vi "AcquireHardware2.vi"(8 "error in (no error)":errorcluster, 11 "SkySparkDevice in":refnum<class "SkySparkDevice.lvclass">) -> (0 "error out":errorcluster, 3 "SkySparkDevice out":refnum<class "SkySparkDevice.lvclass">)   [LabVIEW 2020, in "SkySparkDevice.lvclass"]
uses:
  SkySparkDevice.lvclass
  FGVFunctionTypeDef.ctl
  FGV_TypeDef.ctl
  SkySparkDevice.lvclass/SkySparkDevice.ctl
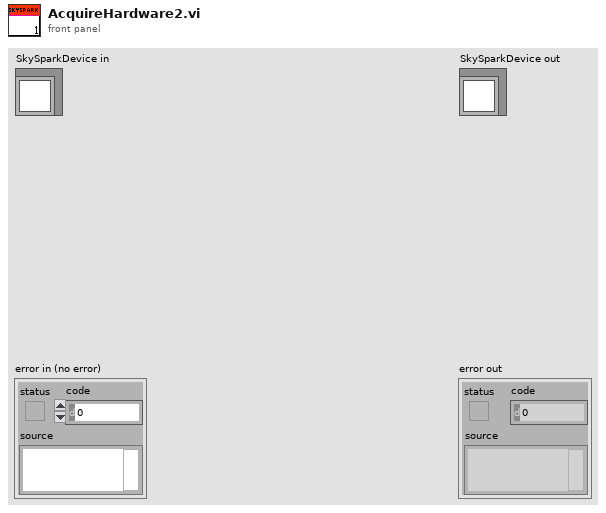
[diagram p1: front panel]
types:
  T1 = typedef "SkySparkDevice.lvclass/FGV_TypeDef.ctl" = cluster{"Data_Array":string[][], "Busy":bool}
  T2 = typedef "SkySparkDevice.lvclass/FGVFunctionTypeDef.ctl" = enum16{"Clear", "Write", "Read"}
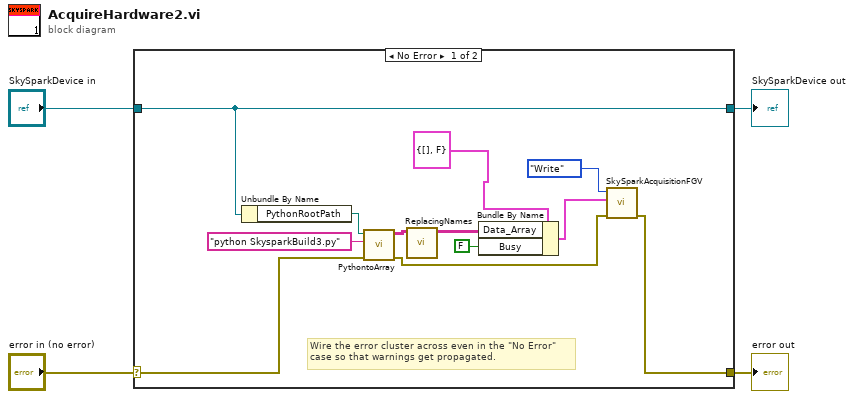
[diagram p0: block diagram]
diagram:
  n1 = case shown="No Error" "error in (no error)" {
    selector: "error in (no error)" -> [w6 w18]
    tunnel: [w5 w18] -> w3
    tunnel: [w8 w17] -> w1
    tunnel: "SkySparkDevice in" -> [w8 w17]
    frame No Error {
      # "Wire the error cluster across even in the \"No Error\"\ncase so that warnings get propagated."
      n2 = Unbundle By Name(w8) -> ("PythonRootPath"=w7:path)
      n3 = call "PythontoArray.vi"("error in (no error)"=w6, "command line"="python SkysparkBuild3.py", "working directory"=w7) -> ("error out"=w10:errorcluster, "Output Array"=w15:string[][])  [unwired: 6 in, 1 out]
      n4 = call "ReplacingNames.vi"("Input Array"=w15) -> ("output array"=w12:string[][])  [unwired: 10 in]
      n5 = Bundle By Name(cluster=T1 {"Data_Array"=[], "Busy"=FALSE} ("FGV_Cluster"), "Data_Array"=w12, "Busy"=FALSE) -> (w11:T1)
      n6 = call "SkySparkAcquisitionFGV.vi"("error in (no error)"=w10, "FGV_Cluster Input"=w11, "Function"=FGVFunctionTypeDef."Write") -> ("error out"=w5:errorcluster)  [unwired: 7 in, 1 out]
    }
    frame Error {
    }
  }
  "error out" <- w3
  "SkySparkDevice out" <- w1
